vi "SCPI Encode.vi"(10 "Arguments [NOUNS]":string[](array[string]), 11 "Command [VERB]":string) -> (3 "Command String":string)   [LabVIEW 2019, in "SCPI.lvclass"]
uses:
  SCPI.lvclass
panel:
  # "Example:\nsetConfig >> Sys >> Time >> hh:mm:ss\nsetConfig >> Sys >> Date >> yyyy:mm:dd\nsetSignal >> Magnet >> Target Current >> float (-170 to +170)\n\nInspiration: SCPI:\n<VERB>:<NOUN>:<NOUN>"
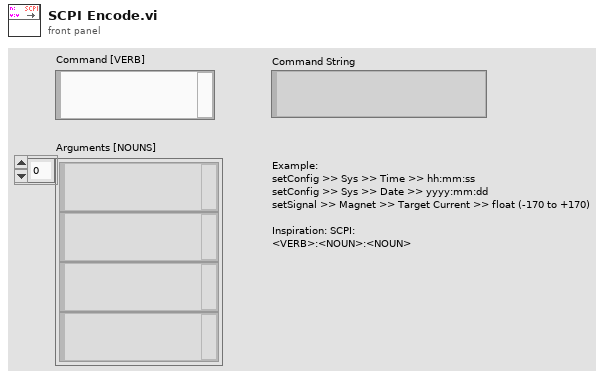
[diagram p1: front panel]
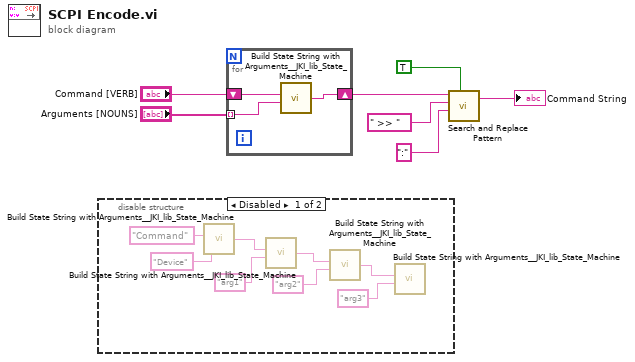
[diagram p0: block diagram]
diagram:
  n1 = disable-structure shown="Disabled" {
    frame Disabled {
      n2 = call <vilib>:"Build State String with Arguments__JKI_lib_State_Machine.vi"("Arguments (\"\")"="Device" ("Arguments (\"\")"), "State"="Command") -> ("State with Arguments"=w15:string)  [unwired: 4 in]
      n3 = call <vilib>:"Build State String with Arguments__JKI_lib_State_Machine.vi"("Arguments (\"\")"="arg1" ("Arguments (\"\")"), "State"=w15) -> ("State with Arguments"=w14:string)  [unwired: 4 in]
      n4 = call <vilib>:"Build State String with Arguments__JKI_lib_State_Machine.vi"("Arguments (\"\")"="arg2" ("Arguments (\"\")"), "State"=w14) -> ("State with Arguments"=w13:string)  [unwired: 4 in]
      n5 = call <vilib>:"Build State String with Arguments__JKI_lib_State_Machine.vi"("Arguments (\"\")"="arg3" ("Arguments (\"\")"), "State"=w13) -> ()  [unwired: 4 in, 1 out]
    }
    frame Enabled {
    }
  }
  n6 = for {
    shift-right: [w16] -> w2
    shift-left: "Command [VERB]" -> [w18]
    tunnel: "Arguments [NOUNS]" -> [w17] mode=indexing
    n7 = call <vilib>:"Build State String with Arguments__JKI_lib_State_Machine.vi"("Arguments (\"\")"=w17, "State"=w18) -> ("State with Arguments"=w16:string)  [unwired: 4 in]
  }
  n8 = call <vilib>:"Search and Replace Pattern.vi"("string"=w2, "regular expression (\"\")"=" >> " ("regular expression (\"\")"), "replace string (\"\")"=":" ("replace string (\"\")"), "replace all? (F)"=TRUE) -> ("result string"=→"Command String":string)  [unwired: 1 in, 1 out]
